vi "数据处理整合 (子VI).vi"(11 "枚举":enum16{"实时数据排序", "小时数据排序"}(ring)) -> (3 "已排序的数组":string[](array[string]))   [LabVIEW 2016, in "数据传输系统.lvlib"]
uses:
  <userlib>/_OpenG.lib/array/array.llb/Remove Duplicates from 1D Array (String)__ogtk.vi
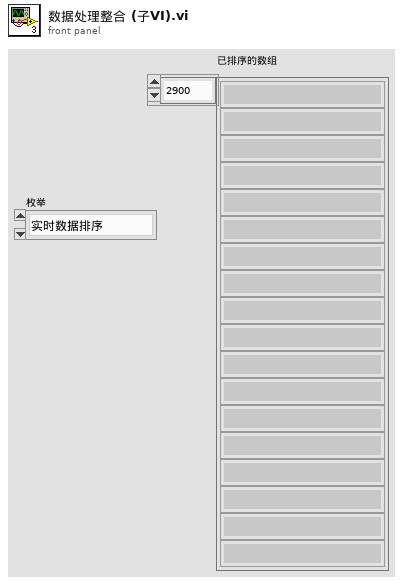
[diagram p1: front panel]
types:
  T1 = cluster{"PH":string[][], "CODCr":string[][], "氨氮":string[][], "CODMn":string[][], "总氮":string[][], "总磷":string[][], "电导率":string[][], "水温":string[][], "DO":string[][], "浊度":string[][], "叶绿素":string[][], "藻密度":string[][], "铜":string[][], "盐度":string[][], "水位":string[][], "流速":string[][], "瞬时流量":string[][], "累积流量":string[][], "亚硝酸盐":string[][], "硫化物":string[][], "ORP":string[][], "铅":string[][], "镉":string[][], "锌":string[][], "镍":string[][], "锰":string[][], "汞":string[][], "气温":string[][], "气压":string[][], "风速":string[][], "风向":string[][]}
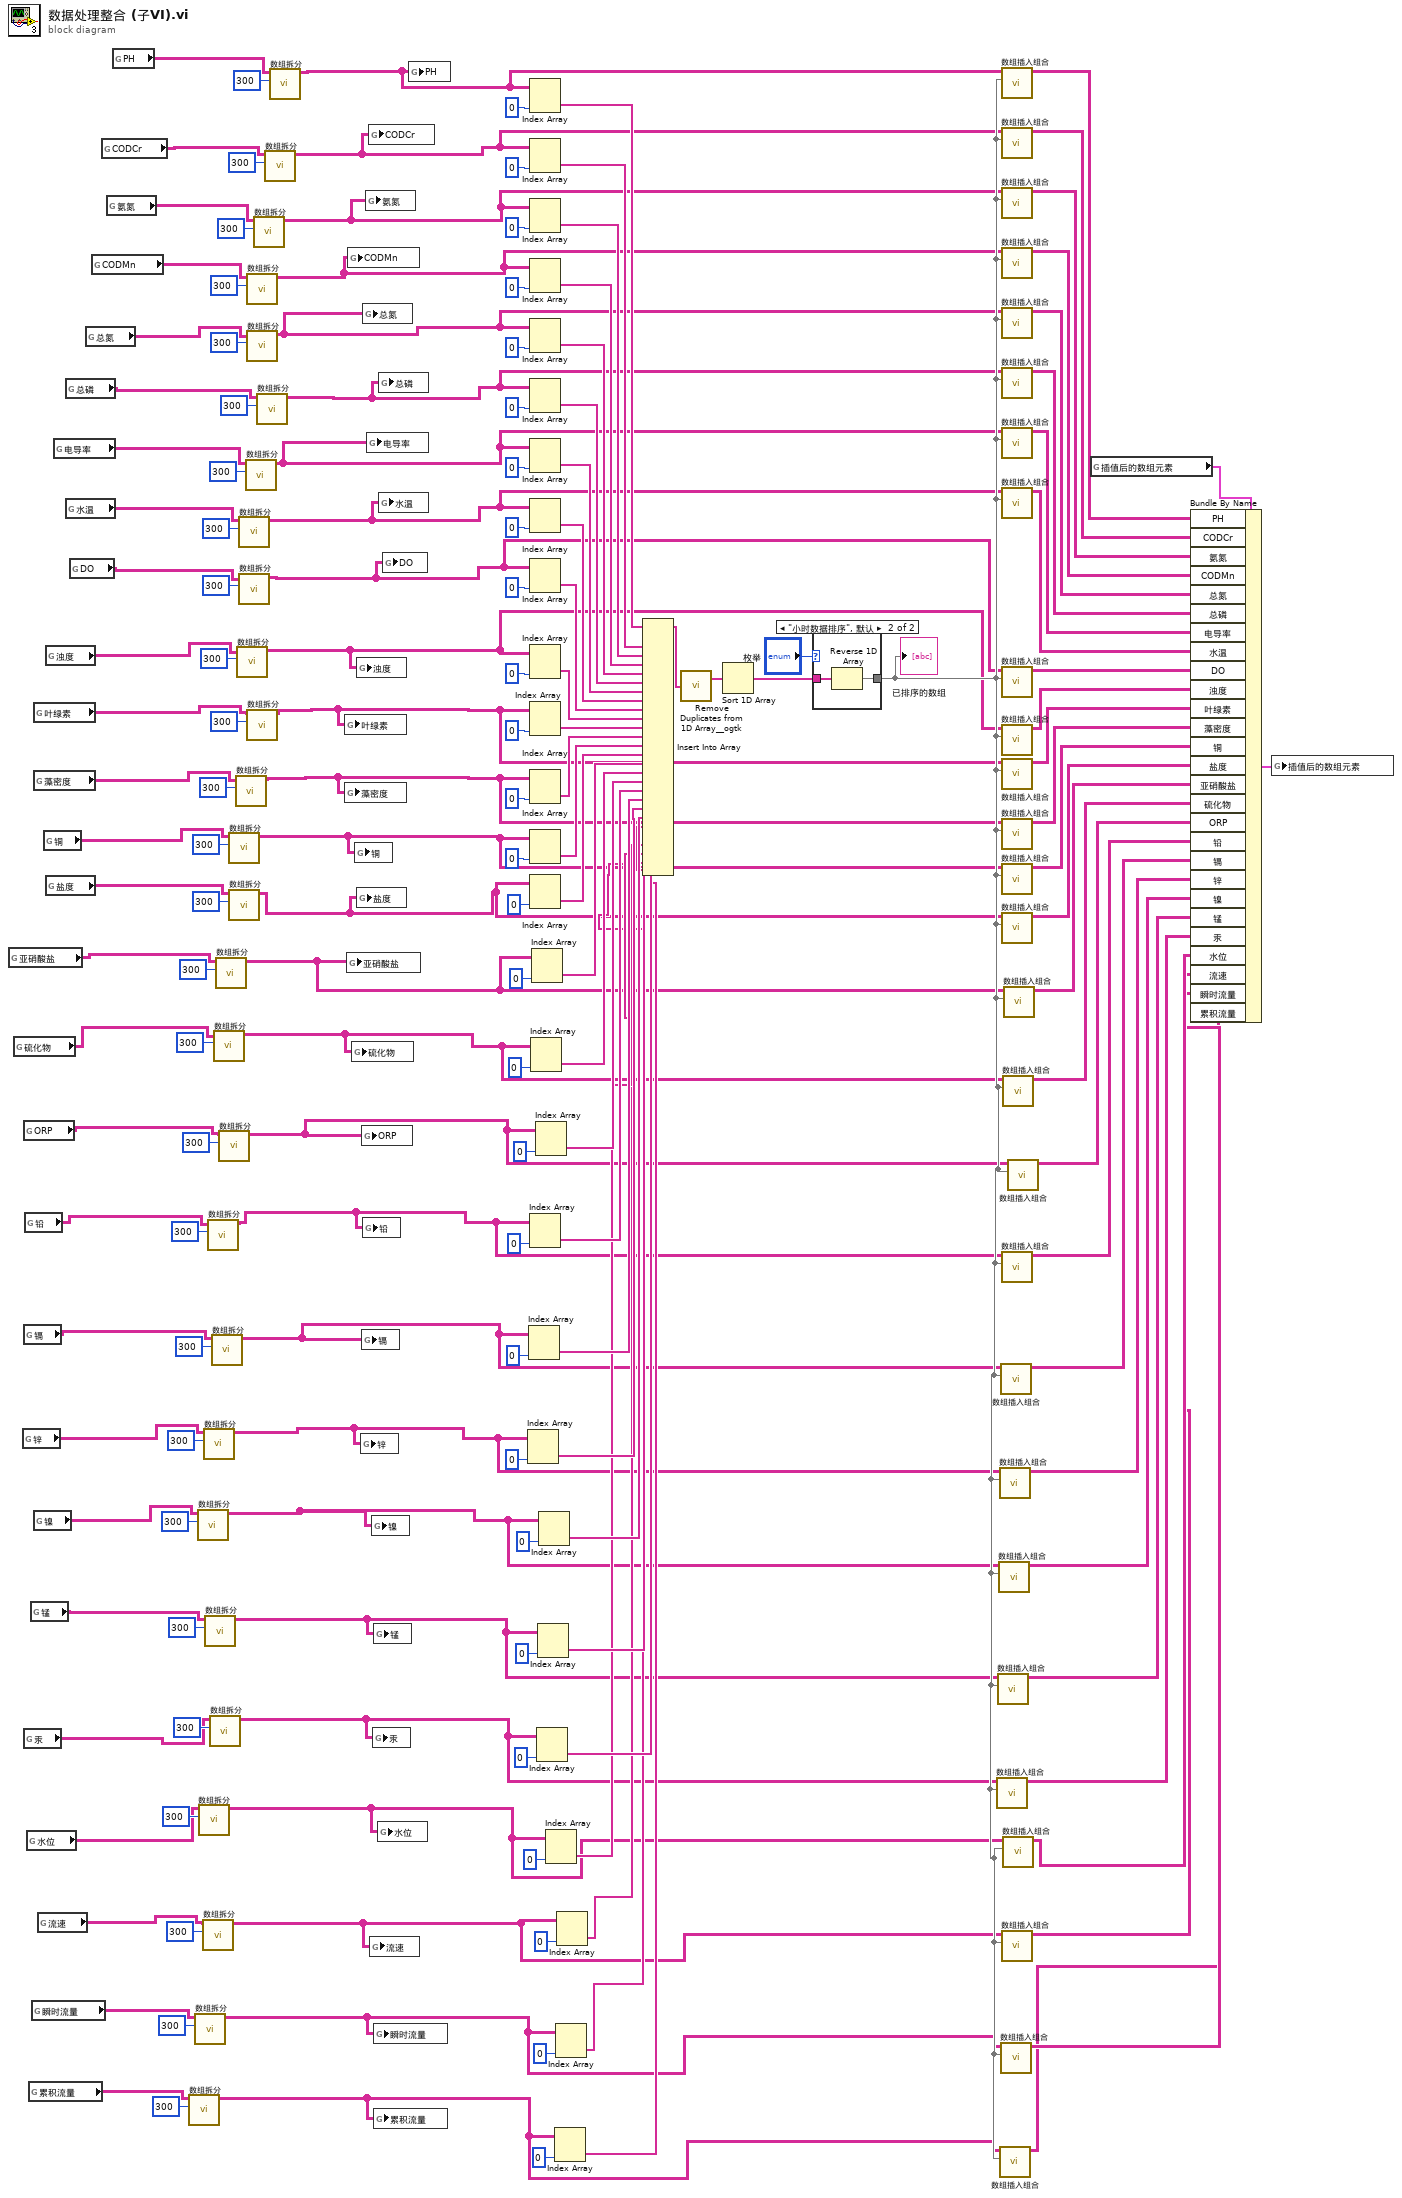
[diagram p0: block diagram]
diagram:
  n1 = global read "全局 所有参数.vi" "亚硝酸盐"() -> (w32:string[][])
  n2 = global read "全局 所有参数.vi" "硫化物"() -> (w31:string[][])
  n3 = global read "全局 所有参数.vi" "锌"() -> (w27:string[][])
  n4 = global read "全局 所有参数.vi" "ORP"() -> (w30:string[][])
  n5 = global read "全局 所有参数.vi" "镉"() -> (w28:string[][])
  n6 = global read "全局 所有参数.vi" "汞"() -> (w11:string[][])
  n7 = global read "全局 所有参数.vi" "铅"() -> (w29:string[][])
  n8 = global read "全局 所有参数.vi" "水位"() -> (w10:string[][])
  n9 = global read "全局 所有参数.vi" "累积流量"() -> (w7:string[][])
  n10 = global read "全局 所有参数.vi" "锰"() -> (w12:string[][])
  n11 = global read "全局 所有参数.vi" "瞬时流量"() -> (w8:string[][])
  n12 = global read "全局 所有参数.vi" "叶绿素"() -> (w48:string[][])
  n13 = global read "全局 所有参数.vi" "藻密度"() -> (w47:string[][])
  n14 = global read "全局 所有参数.vi" "镍"() -> (w26:string[][])
  n15 = global read "全局 所有参数.vi" "流速"() -> (w9:string[][])
  n16 = global read "全局 所有参数.vi" "铜"() -> (w46:string[][])
  n17 = global read "全局 所有参数.vi" "浊度"() -> (w49:string[][])
  n18 = global read "全局 所有参数.vi" "盐度"() -> (w45:string[][])
  n19 = global read "全局 所有参数.vi" "电导率"() -> (w61:string[][])
  n20 = global read "全局 所有参数.vi" "总磷"() -> (w62:string[][])
  n21 = global read "全局 所有参数.vi" "水温"() -> (w60:string[][])
  n22 = global read "全局 所有参数.vi" "DO"() -> (w59:string[][])
  n23 = global read "全局 所有参数.vi" "总氮"() -> (w68:string[][])
  n24 = global read "全局 所有参数.vi" "CODMn"() -> (w71:string[][])
  n25 = global read "全局 所有参数.vi" "CODCr"() -> (w77:string[][])
  n26 = global read "全局 所有参数.vi" "氨氮"() -> (w74:string[][])
  n27 = global read "全局 所有参数.vi" "PH"() -> (w80:string[][])
  n28 = call "数组拆分.vi"("拆分大小"=300, "输入数据"=w7) -> ("输出数组"=w1:string[][])  [unwired: 9 in]
  n29 = call "数组拆分.vi"("拆分大小"=300, "输入数据"=w8) -> ("输出数组"=w2:string[][])  [unwired: 9 in]
  n30 = call "数组拆分.vi"("拆分大小"=300, "输入数据"=w26) -> ("输出数组"=w19:string[][])  [unwired: 9 in]
  n31 = call "数组拆分.vi"("拆分大小"=300, "输入数据"=w10) -> ("输出数组"=w5:string[][])  [unwired: 9 in]
  n32 = call "数组拆分.vi"("拆分大小"=300, "输入数据"=w9) -> ("输出数组"=w3:string[][])  [unwired: 9 in]
  n33 = call "数组拆分.vi"("拆分大小"=300, "输入数据"=w27) -> ("输出数组"=w20:string[][])  [unwired: 9 in]
  n34 = call "数组拆分.vi"("拆分大小"=300, "输入数据"=w12) -> ("输出数组"=w6:string[][])  [unwired: 9 in]
  n35 = call "数组拆分.vi"("拆分大小"=300, "输入数据"=w29) -> ("输出数组"=w22:string[][])  [unwired: 9 in]
  n36 = call "数组拆分.vi"("拆分大小"=300, "输入数据"=w11) -> ("输出数组"=w4:string[][])  [unwired: 9 in]
  n37 = call "数组拆分.vi"("拆分大小"=300, "输入数据"=w28) -> ("输出数组"=w21:string[][])  [unwired: 9 in]
  n38 = call "数组拆分.vi"("拆分大小"=300, "输入数据"=w31) -> ("输出数组"=w24:string[][])  [unwired: 9 in]
  n39 = call "数组拆分.vi"("拆分大小"=300, "输入数据"=w32) -> ("输出数组"=w25:string[][])  [unwired: 9 in]
  n40 = call "数组拆分.vi"("拆分大小"=300, "输入数据"=w30) -> ("输出数组"=w23:string[][])  [unwired: 9 in]
  n41 = call "数组拆分.vi"("拆分大小"=300, "输入数据"=w46) -> ("输出数组"=w42:string[][])  [unwired: 9 in]
  n42 = call "数组拆分.vi"("拆分大小"=300, "输入数据"=w45) -> ("输出数组"=w43:string[][])  [unwired: 9 in]
  n43 = call "数组拆分.vi"("拆分大小"=300, "输入数据"=w47) -> ("输出数组"=w41:string[][])  [unwired: 9 in]
  n44 = call "数组拆分.vi"("拆分大小"=300, "输入数据"=w49) -> ("输出数组"=w44:string[][])  [unwired: 9 in]
  n45 = call "数组拆分.vi"("拆分大小"=300, "输入数据"=w60) -> ("输出数组"=w57:string[][])  [unwired: 9 in]
  n46 = call "数组拆分.vi"("拆分大小"=300, "输入数据"=w59) -> ("输出数组"=w58:string[][])  [unwired: 9 in]
  n47 = call "数组拆分.vi"("拆分大小"=300, "输入数据"=w61) -> ("输出数组"=w56:string[][])  [unwired: 9 in]
  n48 = call "数组拆分.vi"("拆分大小"=300, "输入数据"=w71) -> ("输出数组"=w70:string[][])  [unwired: 9 in]
  n49 = call "数组拆分.vi"("拆分大小"=300, "输入数据"=w68) -> ("输出数组"=w67:string[][])  [unwired: 9 in]
  n50 = call "数组拆分.vi"("拆分大小"=300, "输入数据"=w48) -> ("输出数组"=w40:string[][])  [unwired: 9 in]
  n51 = call "数组拆分.vi"("拆分大小"=300, "输入数据"=w74) -> ("输出数组"=w73:string[][])  [unwired: 9 in]
  n52 = call "数组拆分.vi"("拆分大小"=300, "输入数据"=w62) -> ("输出数组"=w55:string[][])  [unwired: 9 in]
  n53 = call "数组拆分.vi"("拆分大小"=300, "输入数据"=w77) -> ("输出数组"=w76:string[][])  [unwired: 9 in]
  n54 = call "数组拆分.vi"("拆分大小"=300, "输入数据"=w80) -> ("输出数组"=w79:string[][])  [unwired: 9 in]
  n55 = global write "全局 所有参数.vi" "叶绿素"(w40) -> ()
  n56 = global write "全局 所有参数.vi" "藻密度"(w41) -> ()
  n57 = global write "全局 所有参数.vi" "亚硝酸盐"(w25) -> ()
  n58 = global write "全局 所有参数.vi" "CODMn"(w70) -> ()
  n59 = global write "全局 所有参数.vi" "硫化物"(w24) -> ()
  n60 = global write "全局 所有参数.vi" "铜"(w42) -> ()
  n61 = global write "全局 所有参数.vi" "浊度"(w44) -> ()
  n62 = global write "全局 所有参数.vi" "盐度"(w43) -> ()
  n63 = global write "全局 所有参数.vi" "锌"(w20) -> ()
  n64 = global write "全局 所有参数.vi" "ORP"(w23) -> ()
  n65 = global write "全局 所有参数.vi" "镉"(w21) -> ()
  n66 = global write "全局 所有参数.vi" "总氮"(w67) -> ()
  n67 = global write "全局 所有参数.vi" "铅"(w22) -> ()
  n68 = global write "全局 所有参数.vi" "氨氮"(w73) -> ()
  n69 = global write "全局 所有参数.vi" "电导率"(w56) -> ()
  n70 = global write "全局 所有参数.vi" "CODCr"(w76) -> ()
  n71 = global write "全局 所有参数.vi" "流速"(w3) -> ()
  n72 = global write "全局 所有参数.vi" "镍"(w19) -> ()
  n73 = global write "全局 所有参数.vi" "汞"(w4) -> ()
  n74 = global write "全局 所有参数.vi" "锰"(w6) -> ()
  n75 = global write "全局 所有参数.vi" "瞬时流量"(w2) -> ()
  n76 = global write "全局 所有参数.vi" "累积流量"(w1) -> ()
  n77 = global write "全局 所有参数.vi" "水位"(w5) -> ()
  n78 = global write "全局 所有参数.vi" "总磷"(w55) -> ()
  n79 = global write "全局 所有参数.vi" "水温"(w57) -> ()
  n80 = global write "全局 所有参数.vi" "DO"(w58) -> ()
  n81 = global write "全局 所有参数.vi" "PH"(w79) -> ()
  n82 = Index Array(array=w20, index (col)=0 ("索引 (行)")) -> (element=w104:string[])  [unwired: 1 in]
  n83 = Index Array(array=w21, index (col)=0 ("索引 (行)")) -> (element=w105:string[])  [unwired: 1 in]
  n84 = Index Array(array=w79, index (col)=0 ("索引 (行)")) -> (element=w145:string[])  [unwired: 1 in]
  n85 = Index Array(array=w76, index (col)=0 ("索引 (行)")) -> (element=w146:string[])  [unwired: 1 in]
  n86 = Index Array(array=w73, index (col)=0 ("索引 (行)")) -> (element=w147:string[])  [unwired: 1 in]
  n87 = Index Array(array=w70, index (col)=0 ("索引 (行)")) -> (element=w148:string[])  [unwired: 1 in]
  n88 = Index Array(array=w67, index (col)=0 ("索引 (行)")) -> (element=w149:string[])  [unwired: 1 in]
  n89 = Index Array(array=w55, index (col)=0 ("索引 (行)")) -> (element=w150:string[])  [unwired: 1 in]
  n90 = Index Array(array=w56, index (col)=0 ("索引 (行)")) -> (element=w151:string[])  [unwired: 1 in]
  n91 = Index Array(array=w57, index (col)=0 ("索引 (行)")) -> (element=w152:string[])  [unwired: 1 in]
  n92 = Index Array(array=w58, index (col)=0 ("索引 (行)")) -> (element=w153:string[])  [unwired: 1 in]
  n93 = Index Array(array=w44, index (col)=0 ("索引 (行)")) -> (element=w154:string[])  [unwired: 1 in]
  n94 = Index Array(array=w40, index (col)=0 ("索引 (行)")) -> (element=w155:string[])  [unwired: 1 in]
  n95 = Index Array(array=w41, index (col)=0 ("索引 (行)")) -> (element=w156:string[])  [unwired: 1 in]
  n96 = Index Array(array=w42, index (col)=0 ("索引 (行)")) -> (element=w129:string[])  [unwired: 1 in]
  n97 = Index Array(array=w43, index (col)=0 ("索引 (行)")) -> (element=w128:string[])  [unwired: 1 in]
  n98 = Index Array(array=w22, index (col)=0 ("索引 (行)")) -> (element=w106:string[])  [unwired: 1 in]
  n99 = Index Array(array=w24, index (col)=0 ("索引 (行)")) -> (element=w115:string[])  [unwired: 1 in]
  n100 = Index Array(array=w25, index (col)=0 ("索引 (行)")) -> (element=w114:string[])  [unwired: 1 in]
  n101 = Index Array(array=w23, index (col)=0 ("索引 (行)")) -> (element=w116:string[])  [unwired: 1 in]
  n102 = Index Array(array=w4, index (col)=0 ("索引 (行)")) -> (element=w98:string[])  [unwired: 1 in]
  n103 = Index Array(array=w6, index (col)=0 ("索引 (行)")) -> (element=w99:string[])  [unwired: 1 in]
  n104 = Index Array(array=w19, index (col)=0 ("索引 (行)")) -> (element=w100:string[])  [unwired: 1 in]
  n105 = Index Array(array=w5, index (col)=0 ("索引 (行)")) -> (element=w90:string[])  [unwired: 1 in]
  n106 = Index Array(array=w1, index (col)=0 ("索引 (行)")) -> (element=w86:string[])  [unwired: 1 in]
  n107 = Index Array(array=w2, index (col)=0 ("索引 (行)")) -> (element=w87:string[])  [unwired: 1 in]
  n108 = Index Array(array=w3, index (col)=0 ("索引 (行)")) -> (element=w88:string[])  [unwired: 1 in]
  n109 = Insert Into Array(array=w145, new element #1=w146, new element #2=w147, new element #3=w148, new element #4=w149, new element #5=w150, new element #6=w151, new element #7=w152, new element #8=w153, new element #9=w154, new element #10=w155, new element #11=w156, new element #12=w129, new element #13=w128, new element #14=w114, new element #15=w115, new element #16=w116, new element #17=w106, new element #18=w105, new element #19=w104, new element #20=w100, new element #21=w99, new element #22=w98, new element #23=w90, new element #24=w88, new element #25=w87, new element #26=w86) -> (w157:string[])  [unwired: 1 in]
  n110 = call-poly <userlib>:"Remove Duplicates from 1D Array__ogtk.vi"("Input Array"=w157) -> ("Output Array"=w144:string[])  [unwired: 1 out]
  n111 = Sort 1D Array(array=w144) -> (sorted array=w130:string[])
  n112 = case shown="\"小时数据排序\", 默认" "枚举" {
    tunnel: w130 -> [w170 w172]
    tunnel: [w170 w171] -> w89
    frame "实时数据排序" {
    }
    frame "小时数据排序", Default {
      n113 = Reverse 1D Array(array=w172) -> (reversed array=w171:string[])
    }
  }
  "已排序的数组" <- w89
  n114 = call "数组插入组合.vi"("排序后的一维数组"=w89, "输入数组"=w4) -> ("输出结果"=w95:string[][])  [unwired: 9 in]
  n115 = call "数组插入组合.vi"("排序后的一维数组"=w89, "输入数组"=w6) -> ("输出结果"=w96:string[][])  [unwired: 9 in]
  n116 = call "数组插入组合.vi"("排序后的一维数组"=w89, "输入数组"=w19) -> ("输出结果"=w97:string[][])  [unwired: 9 in]
  n117 = call "数组插入组合.vi"("排序后的一维数组"=w89, "输入数组"=w20) -> ("输出结果"=w107:string[][])  [unwired: 9 in]
  n118 = call "数组插入组合.vi"("排序后的一维数组"=w89, "输入数组"=w1) -> ("输出结果"=w82:string[][])  [unwired: 9 in]
  n119 = call "数组插入组合.vi"("排序后的一维数组"=w89, "输入数组"=w21) -> ("输出结果"=w108:string[][])  [unwired: 9 in]
  n120 = call "数组插入组合.vi"("排序后的一维数组"=w89, "输入数组"=w2) -> ("输出结果"=w83:string[][])  [unwired: 9 in]
  n121 = call "数组插入组合.vi"("排序后的一维数组"=w89, "输入数组"=w79) -> ("输出结果"=w158:string[][])  [unwired: 9 in]
  n122 = call "数组插入组合.vi"("排序后的一维数组"=w89, "输入数组"=w76) -> ("输出结果"=w159:string[][])  [unwired: 9 in]
  n123 = call "数组插入组合.vi"("排序后的一维数组"=w89, "输入数组"=w73) -> ("输出结果"=w160:string[][])  [unwired: 9 in]
  n124 = call "数组插入组合.vi"("排序后的一维数组"=w89, "输入数组"=w70) -> ("输出结果"=w161:string[][])  [unwired: 9 in]
  n125 = call "数组插入组合.vi"("排序后的一维数组"=w89, "输入数组"=w67) -> ("输出结果"=w162:string[][])  [unwired: 9 in]
  n126 = call "数组插入组合.vi"("排序后的一维数组"=w89, "输入数组"=w55) -> ("输出结果"=w163:string[][])  [unwired: 9 in]
  n127 = call "数组插入组合.vi"("排序后的一维数组"=w89, "输入数组"=w56) -> ("输出结果"=w164:string[][])  [unwired: 9 in]
  n128 = call "数组插入组合.vi"("排序后的一维数组"=w89, "输入数组"=w57) -> ("输出结果"=w165:string[][])  [unwired: 9 in]
  n129 = call "数组插入组合.vi"("排序后的一维数组"=w89, "输入数组"=w58) -> ("输出结果"=w166:string[][])  [unwired: 9 in]
  n130 = call "数组插入组合.vi"("排序后的一维数组"=w89, "输入数组"=w44) -> ("输出结果"=w167:string[][])  [unwired: 9 in]
  n131 = call "数组插入组合.vi"("排序后的一维数组"=w89, "输入数组"=w40) -> ("输出结果"=w168:string[][])  [unwired: 9 in]
  n132 = call "数组插入组合.vi"("排序后的一维数组"=w89, "输入数组"=w41) -> ("输出结果"=w169:string[][])  [unwired: 9 in]
  n133 = call "数组插入组合.vi"("排序后的一维数组"=w89, "输入数组"=w42) -> ("输出结果"=w127:string[][])  [unwired: 9 in]
  n134 = call "数组插入组合.vi"("排序后的一维数组"=w89, "输入数组"=w43) -> ("输出结果"=w126:string[][])  [unwired: 9 in]
  n135 = call "数组插入组合.vi"("排序后的一维数组"=w89, "输入数组"=w22) -> ("输出结果"=w109:string[][])  [unwired: 9 in]
  n136 = call "数组插入组合.vi"("排序后的一维数组"=w89, "输入数组"=w3) -> ("输出结果"=w84:string[][])  [unwired: 9 in]
  n137 = call "数组插入组合.vi"("排序后的一维数组"=w89, "输入数组"=w24) -> ("输出结果"=w117:string[][])  [unwired: 9 in]
  n138 = call "数组插入组合.vi"("排序后的一维数组"=w89, "输入数组"=w5) -> ("输出结果"=w85:string[][])  [unwired: 9 in]
  n139 = call "数组插入组合.vi"("排序后的一维数组"=w89, "输入数组"=w25) -> ("输出结果"=w119:string[][])  [unwired: 9 in]
  n140 = call "数组插入组合.vi"("排序后的一维数组"=w89, "输入数组"=w23) -> ("输出结果"=w118:string[][])  [unwired: 9 in]
  n141 = global read "插值后的新数组.vi" "插值后的数组元素"() -> (w123:T1)
  n142 = Bundle By Name(cluster=w123, "PH"=w158, "CODCr"=w159, "氨氮"=w160, "CODMn"=w161, "总氮"=w162, "总磷"=w163, "电导率"=w164, "水温"=w165, "DO"=w166, "浊度"=w167, "叶绿素"=w168, "藻密度"=w169, "铜"=w127, "盐度"=w126, "亚硝酸盐"=w119, "硫化物"=w117, "ORP"=w118, "铅"=w109, "镉"=w108, "锌"=w107, "镍"=w97, "锰"=w96, "汞"=w95, "水位"=w85, "流速"=w84, "瞬时流量"=w83, "累积流量"=w82) -> (w113:T1)
  n143 = global write "插值后的新数组.vi" "插值后的数组元素"(w113) -> ()
